vi "Gyro Signal 3-Axis Display from Control MCU.vi"() -> ()   [LabVIEW 2015]
uses:
  <vilib>/Utility/error.llb/DialogType.ctl
  <vilib>/Instr/_visa.llb/VISA Configure Serial Port (Instr).vi
panel:
  out "Numeric":dbl=1.0
  out "return count":u32
  in  "Start/Stop \nTracking":bool
  in  "Cluster":T1
  out "System Time":dbl
  in  "Stop Button":bool
  out "Gyro Reading Z":dbl(knob) scale=-250.0..250.0
  out "Gyro Reading Y":dbl(knob) scale=-250.0..250.0
  out "Data Buffer":u8[](array[numeric])
  in  "parity (0:none)":enum16{"None", "Odd", "Even", "Mark", "Space"}(ring)
  out "Gyro Reading X":dbl(knob) scale=-250.0..250.0
  in  "VISA resource name":refnum<visa-resource-name>="COM5"
  in  "Stop bits (1 bit)":u16(ring)=10 items=["1.0"=10, "1.5"=15, "2.0"=20]
  in  "Baud rate":u32=115200
  # "Setup of Basic Serial Coms"
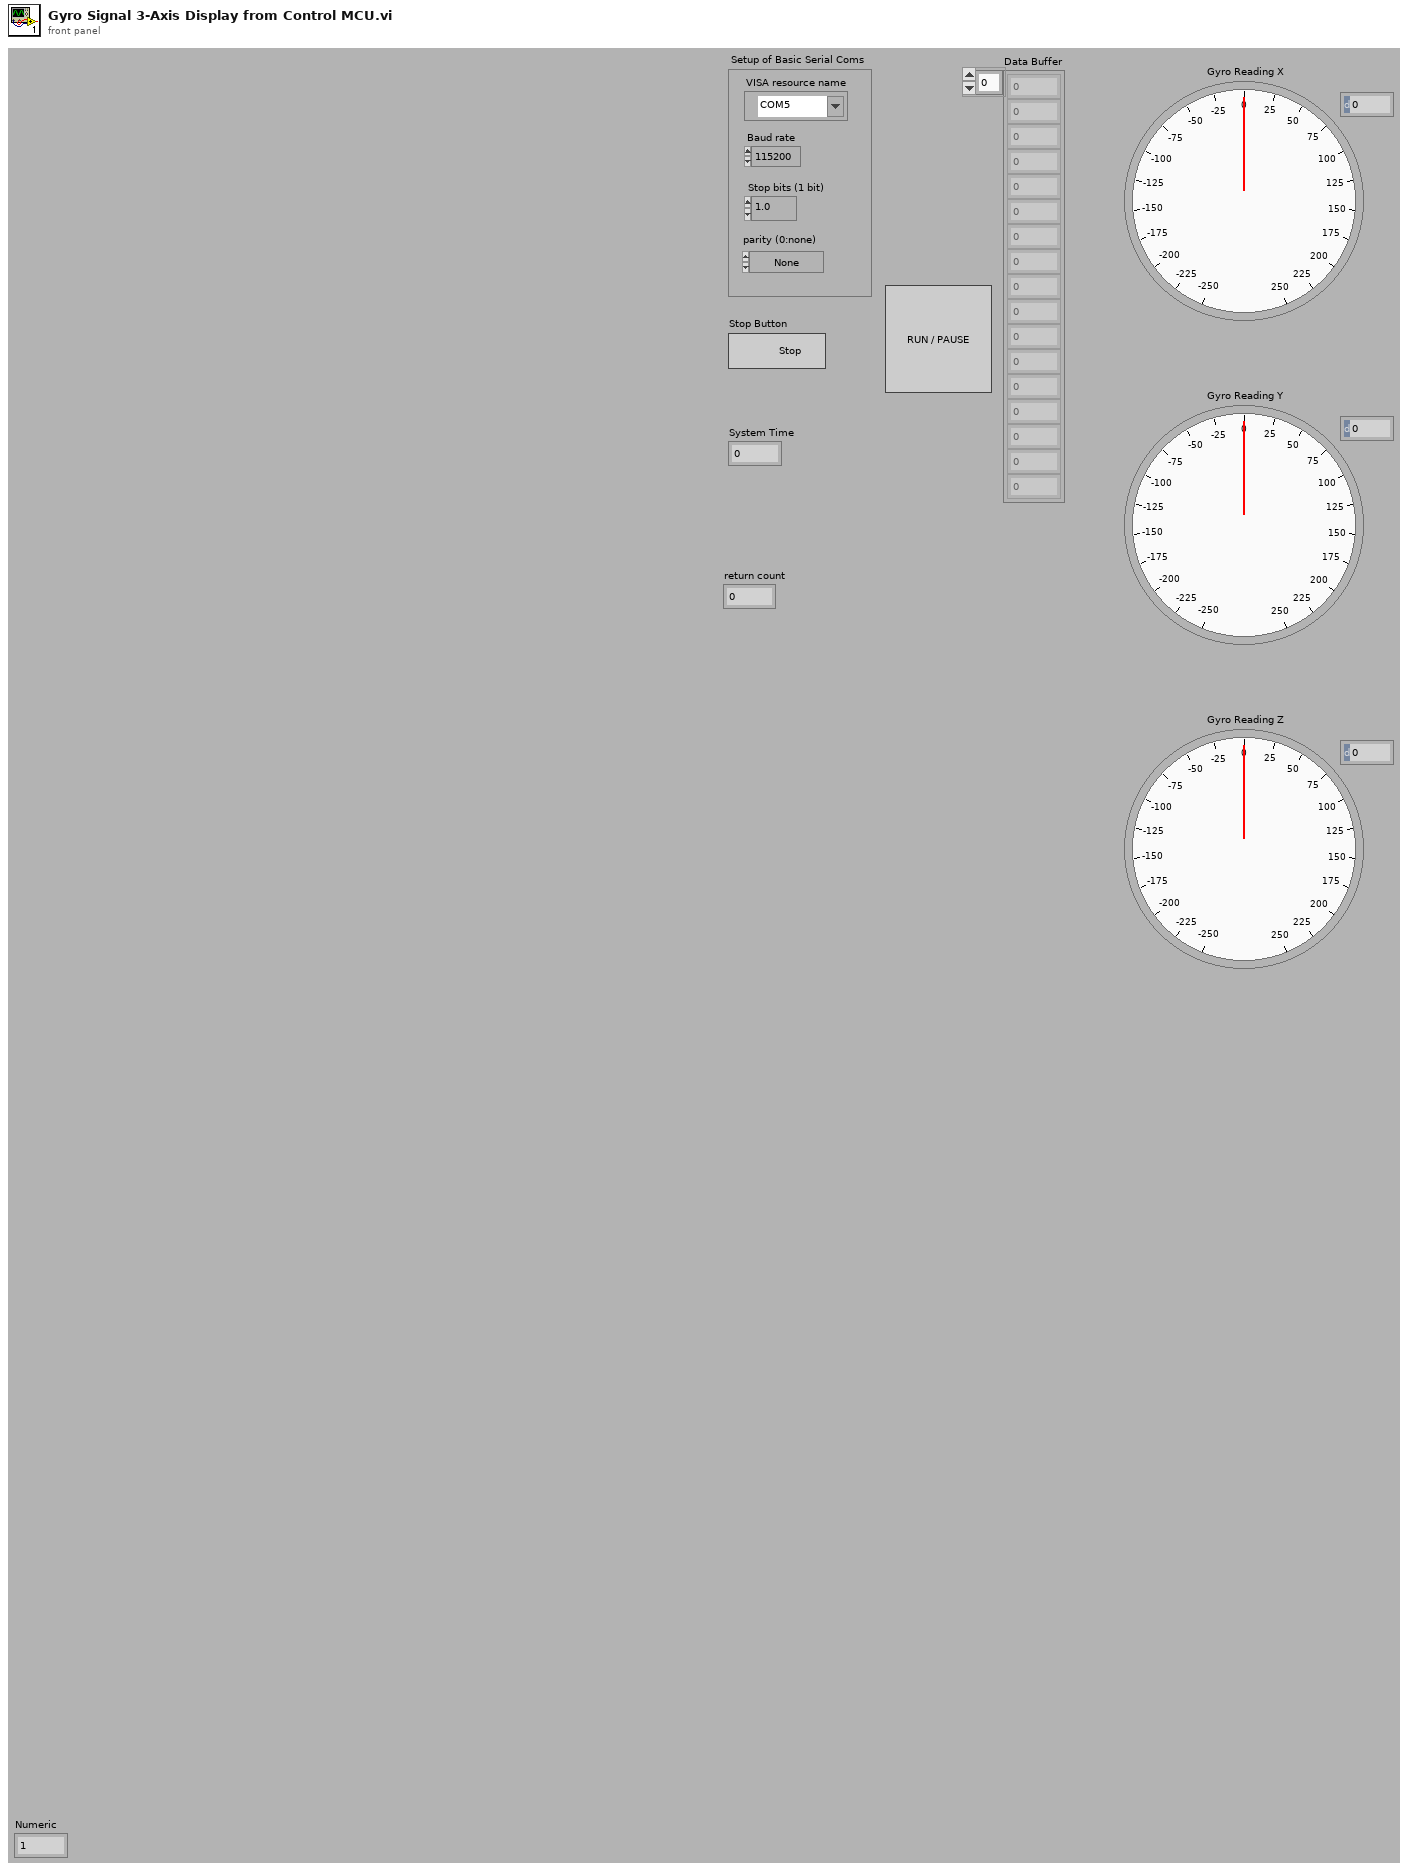
[diagram p1: front panel]
types:
  T1 = cluster{"X":dbl[], "Y":dbl[], "Z":dbl[], "theta":u16[], "phi":u16[], "CX":u16[], "CY":u16[], "Time":dbl[]}
  T2 = typedef "DialogType.ctl" = u16
  T3 = cluster{dbl[], dbl[], dbl[], u16[], u16[], u16[], u16[], dbl[]}
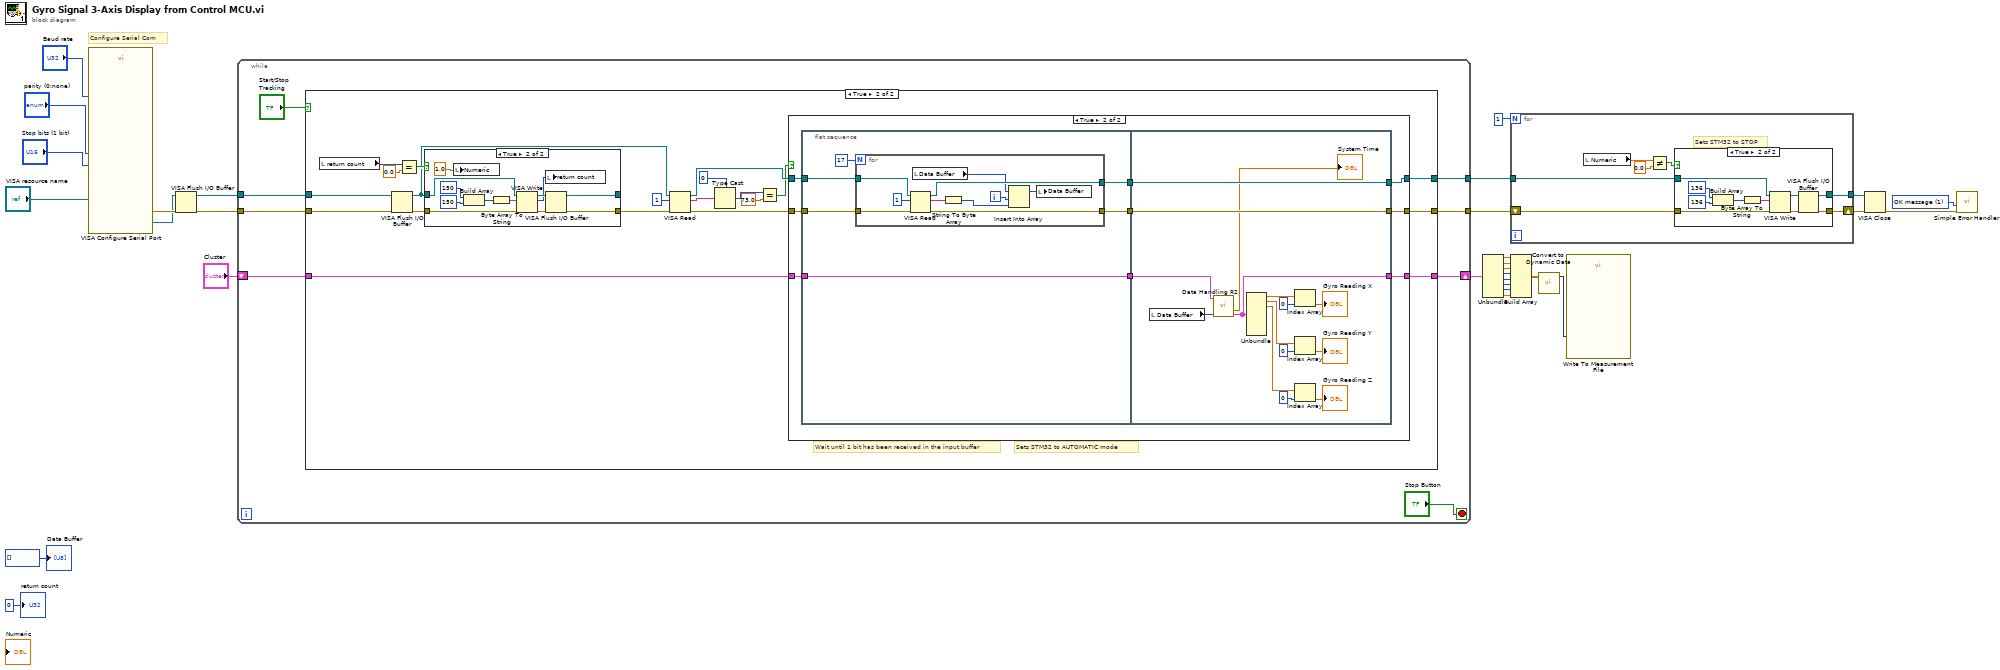
[diagram p0: block diagram]
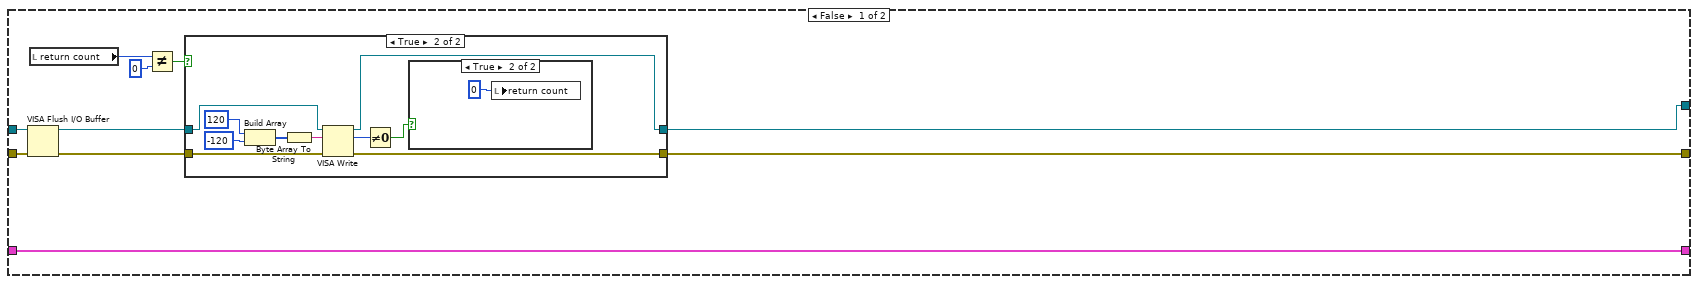
[diagram p3: hidden frame]
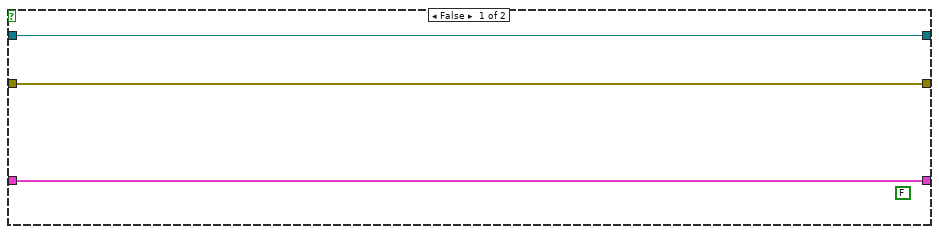
[diagram p7: hidden frame]
diagram:
  w25 = T2 1 items=["no dialog", "OK message", "continue or stop message", "OK message + warnings", "continue/stop + warnings"] ("type of dialog (OK msg:1)")
  # "Configure Serial Com"
  n1 = call-poly "VISA Configure Serial Port"("VISA resource name"="VISA resource name", "baud rate (9600)"="Baud rate", "parity (0:none)"="parity (0:none)", "stop bits (10: 1 bit)"="Stop bits (1 bit)") -> ("VISA resource name out"=w23:refnum<visa-resource-name>, "error out"=w24:errorcluster)  [unwired: 10 in]
  n2 = VISA Flush I/O Buffer(VISA resource name=w23, error in (no error)=w24) -> (VISA resource name out=w22:refnum<visa-resource-name>, error out=w21:errorcluster)  [unwired: 1 in]
  n3 = while {
    tunnel: w22 -> [w35]
    tunnel: w21 -> [w34]
    tunnel: [w37] -> w3
    tunnel: [w36] -> w2
    shift-right: [w32] -> w7
    shift-left: "Cluster" -> [w31]
    stop <- "Stop Button" stop-if-true
    n4 = case shown="True" "Start/Stop \nTracking" {
      tunnel: [w40 w80] -> w37
      tunnel: [w39 w79] -> w36
      tunnel: w35 -> [w42 w63]
      tunnel: w34 -> [w41 w62]
      tunnel: [w38 w70] -> w32
      tunnel: w31 -> [w38 w69]
      frame False {
        n5 = VISA Flush I/O Buffer(VISA resource name=w42, error in (no error)=w41) -> (VISA resource name out=w44:refnum<visa-resource-name>, error out=w43:errorcluster)  [unwired: 1 in]
        n6 = local read "return count"() -> (w47:u32)
        n7 = Not Equal?(x=w47, y=u32 0) -> (x != y?=w45:bool)
        n8 = case shown="True" w45 {
          tunnel: w44 -> [w49 w59]
          tunnel: w43 -> [w48 w58]
          tunnel: [w49 w57] -> w40
          tunnel: [w48 w56] -> w39
          frame False {
          }
          frame True {
            n9 = Build Array(i8 120 ("element"), i8 -120 ("element")) -> (w52:i8[])
            n10 = Byte Array To String(unsigned byte array=w52) -> (string=w55:string)
            n11 = VISA Write(VISA resource name=w59, write buffer=w55, error in (no error)=w58) -> (VISA resource name out=w57:refnum<visa-resource-name>, return count=w50:u32, error out=w56:errorcluster)
            n12 = Not Equal To 0?(x=w50) -> (x != 0?=w51:bool)
            n13 = case shown="True" w51 {
              frame False {
              }
              frame True {
                n14 = local write "return count"(u32 0 ("return count")) -> ()
              }
            }
          }
        }
      }
      frame True {
        # "Sets STM32 to AUTOMATIC mode"
        # "Wait until 1 bit has been received in the input buffer"
        n15 = local read "return count"() -> (w61:u32)
        n16 = VISA Flush I/O Buffer(VISA resource name=w63, error in (no error)=w62) -> (VISA resource name out=w65:refnum<visa-resource-name>, error out=w66:errorcluster)  [unwired: 1 in]
        n17 = Equal?(x=w61, y=0.0) -> (x = y?=w68:bool)
        n18 = case shown="True" w68 {
          tunnel: w65 -> [w82 w90]
          tunnel: w66 -> [w81 w89]
          tunnel: [w82 w86] -> _
          tunnel: [w81 w85] -> w64
          frame False {
          }
          frame True {
            n19 = local write "Numeric"(1.0 ("Numeric")) -> ()
            n20 = Build Array(u8 150 ("element"), u8 150 ("element")) -> (w91:u8[])
            n21 = Byte Array To String(unsigned byte array=w91) -> (string=w94:string)
            n22 = VISA Write(VISA resource name=w90, write buffer=w94, error in (no error)=w89) -> (VISA resource name out=w88:refnum<visa-resource-name>, return count=w83:u32, error out=w87:errorcluster)
            n23 = local write "return count"(w83) -> ()
            n24 = VISA Flush I/O Buffer(VISA resource name=w88, error in (no error)=w87) -> (VISA resource name out=w86:refnum<visa-resource-name>, error out=w85:errorcluster)  [unwired: 1 in]
          }
        }
        n25 = VISA Read(VISA resource name=w65, byte count=u32 1, error in (no error)=w64) -> (VISA resource name out=w77:refnum<visa-resource-name>, read buffer=w71:string, error out=w76:errorcluster)  [unwired: 1 out]
        n26 = Type Cast(type=u8 0, x=w71) -> (*(type *) &x=w74:u8)
        n27 = Equal?(x=w74, y=73.0) -> (x = y?=w72:bool)
        n28 = case shown="True" w72 {
          tunnel: [w97 w104] -> w80
          tunnel: [w96 w103] -> w79
          tunnel: w77 -> [w97 w102]
          tunnel: w76 -> [w96 w101]
          tunnel: w69 -> [w95 w99]
          tunnel: [w95 w98] -> w70
          frame False {
            (unwired) FALSE ("LIMIT ERROR")
          }
          frame True {
            n29 = flat-sequence {
              tunnel: [w111] -> w106
              tunnel: [w110] -> w105
              tunnel: w102 -> [w109]
              tunnel: w101 -> [w108]
              tunnel: [w107] -> w100
              tunnel: w99 -> [w107]
              tunnel: w106 -> [w137]
              tunnel: w105 -> [w136]
              tunnel: [w137] -> w104
              tunnel: [w136] -> w103
              tunnel: w100 -> [w134]
              tunnel: [w126] -> w98
              frame #0 {
                n30 = for {
                  N: 17 -> [_]
                  tunnel: [w121] -> w111
                  tunnel: [w120] -> w110
                  tunnel: w109 -> [w114]
                  tunnel: w108 -> [w113]
                  i -> [w115]
                  n31 = VISA Read(VISA resource name=w114, byte count=u32 1, error in (no error)=w113) -> (VISA resource name out=w121:refnum<visa-resource-name>, read buffer=w119:string, error out=w120:errorcluster)  [unwired: 1 out]
                  n32 = local read "Data Buffer"() -> (w117:u8[])
                  n33 = String To Byte Array(string=w119) -> (unsigned byte array=w118:u8[])
                  n34 = Insert Into Array(array=w117, index=w115, new element=w118) -> (w116:u8[])
                  n35 = local write "Data Buffer"(w116) -> ()
                }
              }
              frame #1 {
                n36 = local read "Data Buffer"() -> (w135:u8[])
                n37 = call "Data Handling R2.vi"("Cluster"=w134, "Data Buffer"=w135) -> ("Time"=→"System Time":dbl, "output cluster"=w126:T3)  [unwired: 5 in, 7 out]
                n38 = Unbundle(w126) -> (w129:dbl[], w128:dbl[], w127:dbl[])  [unwired: 5 out]
                n39 = Index Array(array=w129, index=0) -> (element=→"Gyro Reading X":dbl)
                n40 = Index Array(array=w128, index=0) -> (element=→"Gyro Reading Y":dbl)
                n41 = Index Array(array=w127, index=0) -> (element=→"Gyro Reading Z":dbl)
              }
            }
          }
        }
      }
    }
  }
  n42 = Unbundle(w7) -> ("X"=w17:dbl[], "Y"=w16:dbl[], "Z"=w15:dbl[], "theta"=w14:u16[], "phi"=w13:u16[], "CX"=w12:u16[], "CY"=w11:u16[], "Time"=w8:dbl[])
  n43 = for {
    N: 1 -> [_]
    tunnel: w3 -> [w142]
    shift-right: [w139] -> w4
    shift-left: w2 -> [w141]
    tunnel: [w138] -> w5
    # "Sets STM32 to STOP"
    n44 = local read "Numeric"() -> (w140:dbl)
    n45 = Not Equal?(x=w140, y=0.0) -> (x != y?=w143:bool)
    n46 = case shown="True" w143 {
      tunnel: [w146 w148] -> w139
      tunnel: w142 -> [w145 w152]
      tunnel: w141 -> [w146 w151]
      tunnel: [w145 w147] -> w138
      frame False {
      }
      frame True {
        n47 = Build Array(u8 136 ("element"), u8 136 ("element")) -> (w153:u8[])
        n48 = Byte Array To String(unsigned byte array=w153) -> (string=w156:string)
        n49 = VISA Write(VISA resource name=w152, write buffer=w156, error in (no error)=w151) -> (VISA resource name out=w150:refnum<visa-resource-name>, error out=w149:errorcluster)  [unwired: 1 out]
        n50 = VISA Flush I/O Buffer(VISA resource name=w150, error in (no error)=w149) -> (VISA resource name out=w147:refnum<visa-resource-name>, error out=w148:errorcluster)  [unwired: 1 in]
      }
    }
  }
  n51 = Build Array(w17, w16, w15, w14, w13, w12, w11, w8) -> (w10:dbl[][])
  n52 = call "Convert to Dynamic Data"("2D Array"=w10) -> ("Dynamic Data Type"=w9:dynamicdata)  [unwired: 3 in]
  n53 = call "Write To Measurement File"("Signals"=w9) -> ()  [unwired: 16 in, 3 out]
  n54 = VISA Close(VISA resource name=w5, error in (no error)=w4) -> (error out=w26:errorcluster)
  n55 = call <vilib>:"Simple Error Handler.vi"("type of dialog (OK msg:1)"=w25, "error in (no error)"=w26) -> ()  [unwired: 3 in, 5 out]
  "Data Buffer" <- u8[] [] ("Data Buffer")
  "return count" <- u32 0 ("return count")
